vi "Main.vi"() -> ()   [LabVIEW 2015]
uses:
  TypDefs/Loop States.ctl
  TypDefs/Loop Data.ctl
panel:
  in  "device name":tag="myDAQ1"
  in  "Exit Button":bool
  in  "Start Button":bool
  out "Status":string
  in  "Clear Button":bool
  in  "Save Button":bool
  out "XY Graph":cluster{"X":dbl[], "Y":dbl[]}(graph)
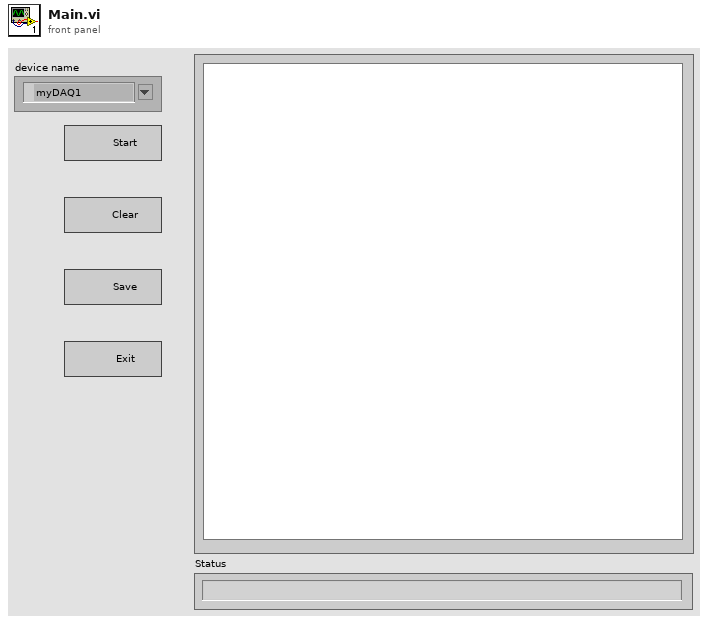
[diagram p1: front panel]
types:
  T1 = typedef "Loop Data.ctl" = cluster{"Status":string, "Graph Data":cluster{"X":dbl[], "Y":dbl[]}, "Recording Status":bool}
  T2 = typedef "Loop States.ctl" = enum16{"Error", "Wait for events", "Measure positions", "Update UI", "Initialization"}
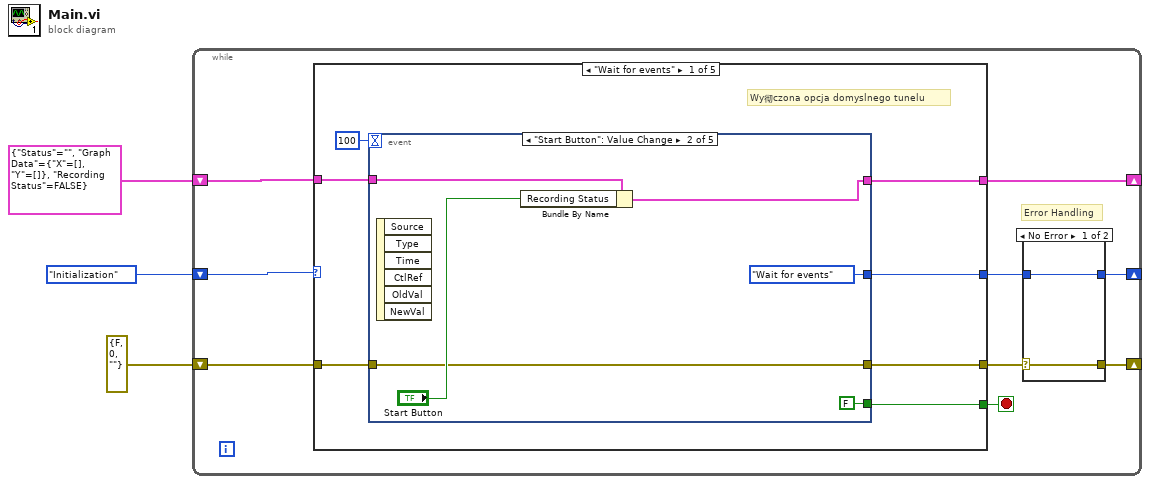
[diagram p0: block diagram]
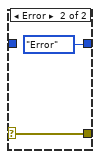
[diagram p2: hidden frame]
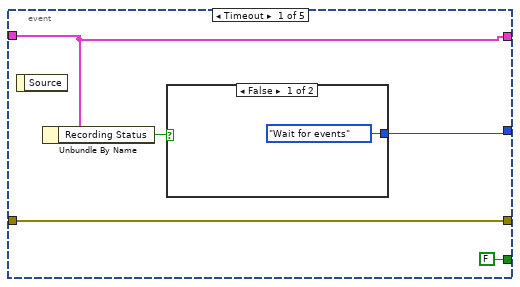
[diagram p3: hidden frame]
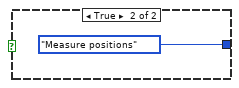
[diagram p4: hidden frame]
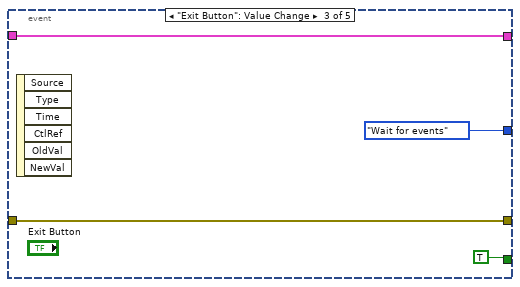
[diagram p5: hidden frame]
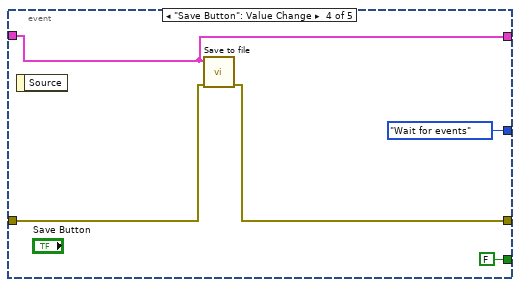
[diagram p6: hidden frame]
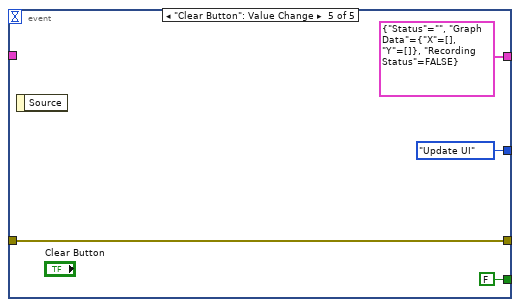
[diagram p7: hidden frame]
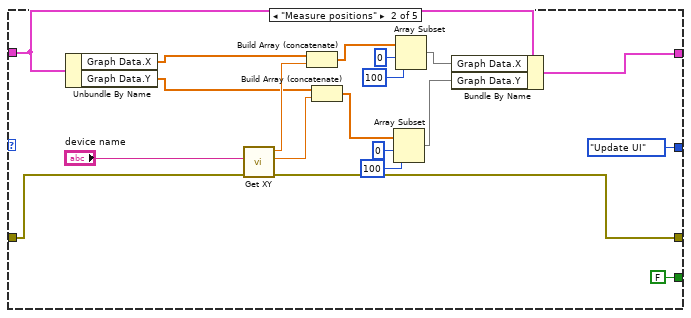
[diagram p8: hidden frame]
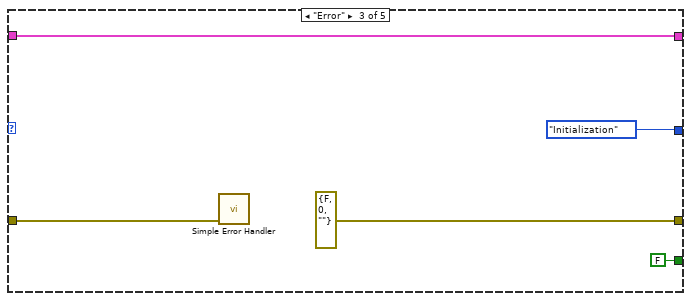
[diagram p9: hidden frame]
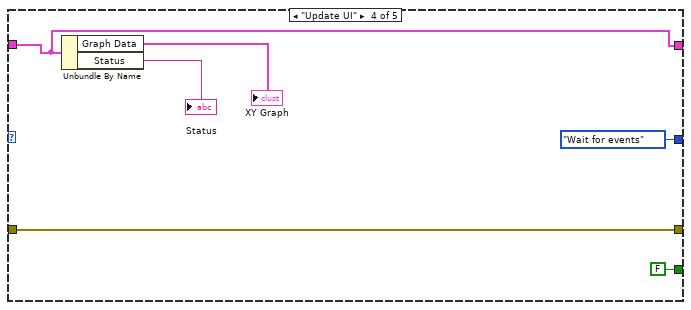
[diagram p10: hidden frame]
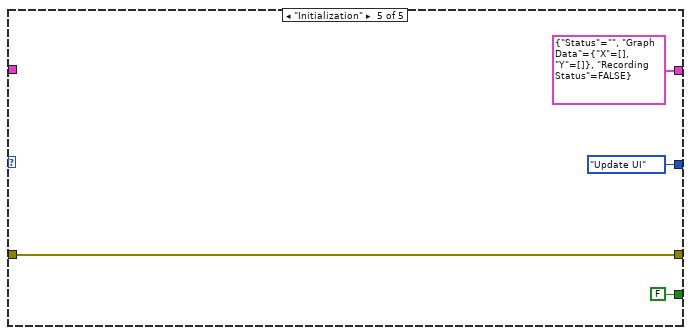
[diagram p11: hidden frame]
diagram:
  n1 = while {
    shift-right: [w10] -> _
    shift-left: T1 {"Status"="", "Graph Data"={"X"=[], "Y"=[]}, "Recording Status"=FALSE} -> [w11]
    shift-right: [w5] -> _
    shift-left: Loop_States."Initialization" -> [w12]
    shift-right: [w4] -> _
    shift-left: errorcluster {"status"=FALSE, "code"=0, "source"=""} ("error constant") -> [w8]
    stop <- w9 stop-if-true
    # "Error Handling"
    n2 = case shown="\"Wait for events\"" w12 {
      tunnel: w11 -> [w22 w65 w70 w75 _]
      tunnel: [w20 w67 w70 w75 T1 {"Status"="", "Graph Data"={"X"=[], "Y"=[]}, "Recording Status"=FALSE}] -> w10
      tunnel: [w19 FALSE FALSE FALSE FALSE] -> w9
      tunnel: [w21 Loop_States."Update UI" Loop_States."Initialization" Loop_States."Wait for events" Loop_States."Update UI"] -> w6
      tunnel: w8 -> [w18 w63 w72 w78 w81]
      tunnel: [w17 w64 errorcluster {"status"=FALSE, "code"=0, "source"=""} ("error constant") w78 w81] -> w7
      frame "Wait for events" {
        # "Wy彻czona opcja domyslnego tunelu"
        n3 = event shown="[1] \"Start Button\": Value Change" {
          selector: _ -> [_ _ _ _ _]
          dyn-events: _ -> [_ _ _ _ _]
          timeout: 100 -> [_ _ _ _ _]
          tunnel: w22 -> [w25 w36 w39 w42 _]
          tunnel: [w24 Loop_States."Wait for events" Loop_States."Wait for events" Loop_States."Wait for events" Loop_States."Update UI"] -> w21
          tunnel: [w25 w34 w39 w42 T1 {"Status"="", "Graph Data"={"X"=[], "Y"=[]}, "Recording Status"=FALSE}] -> w20
          tunnel: [FALSE FALSE TRUE FALSE FALSE] -> w19
          tunnel: w18 -> [w28 w32 w37 w44 w47]
          tunnel: [w28 w32 w37 w43 w47] -> w17
          event Timeout {
            n4 = event-data() -> ()  [unwired: 1 in, 1 out]
            n5 = Unbundle By Name(w25) -> ("Recording Status"=w26:bool)
            n6 = case shown="False" w26 {
              tunnel: [Loop_States."Wait for events" Loop_States."Measure positions"] -> w24
              frame False {
              }
              frame True {
              }
            }
          }
          event "Start Button": Value Change {
            n7 = event-data() -> ()  [unwired: 1 in, 6 out]
            n8 = Bundle By Name(cluster=w36, "Recording Status"="Start Button") -> (w34:T1)
          }
          event "Exit Button": Value Change {
            n9 = event-data() -> ()  [unwired: 1 in, 6 out]
          }
          event "Save Button": Value Change {
            n10 = event-data() -> ()  [unwired: 1 in, 1 out]
            n11 = call "Save to file.vi"("error in (no error)"=w44, "Loop Data"=w42) -> ("error out"=w43:errorcluster)  [unwired: 9 in]
          }
          event "Clear Button": Value Change {
            n12 = event-data() -> ()  [unwired: 1 in, 1 out]
          }
        }
      }
      frame "Measure positions" {
        n13 = Unbundle By Name(w65) -> ("Graph Data.X"=w61:dbl[], "Graph Data.Y"=w59:dbl[])
        n14 = call "Get XY.vi"("error in"=w63, "device name"="device name") -> ("error out"=w64:errorcluster, "Y"=w58:dbl, "X"=w60:dbl)  [unwired: 7 in]
        n15 = Build Array (concatenate)(w61, w60) -> (w57:dbl[])
        n16 = Build Array (concatenate)(w59, w58) -> (w55:dbl[])
        n17 = Array Subset(array=w55, index=0, length=100) -> (w54:dbl[])
        n18 = Array Subset(array=w57, index=0, length=100) -> (w56:dbl[])
        n19 = Bundle By Name(cluster=w65, "Graph Data.X"=w56, "Graph Data.Y"=w54) -> (w67:T1)
      }
      frame "Error" {
        n20 = call <vilib>:"Simple Error Handler.vi"("error in (no error)"=w72) -> ()  [unwired: 4 in, 5 out]
      }
      frame "Update UI" {
        n21 = Unbundle By Name(w75) -> ("Graph Data"=→"XY Graph":cluster{"X":dbl[], "Y":dbl[]}, "Status"=→"Status":string)
      }
      frame "Initialization" {
      }
    }
    n22 = case shown="No Error" w7 {
      selector: w7 -> [w13 w15]
      tunnel: w6 -> [w14 _]
      tunnel: [w14 Loop_States."Error"] -> w5
      tunnel: [w13 w15] -> w4
      frame No Error {
      }
      frame Error {
      }
    }
  }
